vi "wait_with_status.vi"(4 "stat ref":refnum<vi>, 6 "stop ref":refnum<vi>, 7 "second stop ref":refnum<vi>, 8 "error in":errorcluster, 9 "comment":string, 10 "ignore error (False)":bool, 11 "ms to wait":i32) -> (0 "error out":errorcluster, 2 "Aborted?":bool)   [LabVIEW 2020, in "varilib.lvlib"]
doc: "Interruptable delay timer. It waits for given amount of milliseconds. When 'stop ref' is assigned with reference to boolean button it will terminate the delay when logical state of the boolean is True. If 'stat ref' is assigned with reference to string indicator and delay is over 1 second it will periodically write status string in following format:'Waiting 3 of 10 seconds%s' where %s is content of 'comment' input. When the wait loop is done the original content of 'stat ref' will be restored.\nThe second reference control is used to interrupt delay, however control is fully controlled by this VI: showing, reading and setting state, hiding."
uses:
  varilib.lvlib
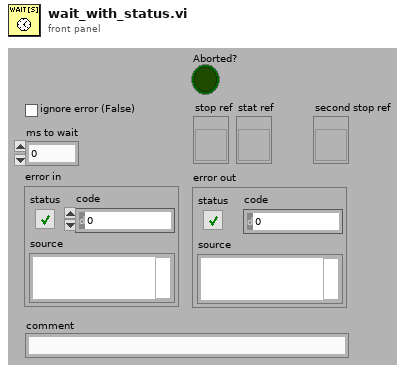
[diagram p1: front panel]
types:
  T1 = enum8{"Enabled", "Disabled", "Disabled and Grayed Out"}
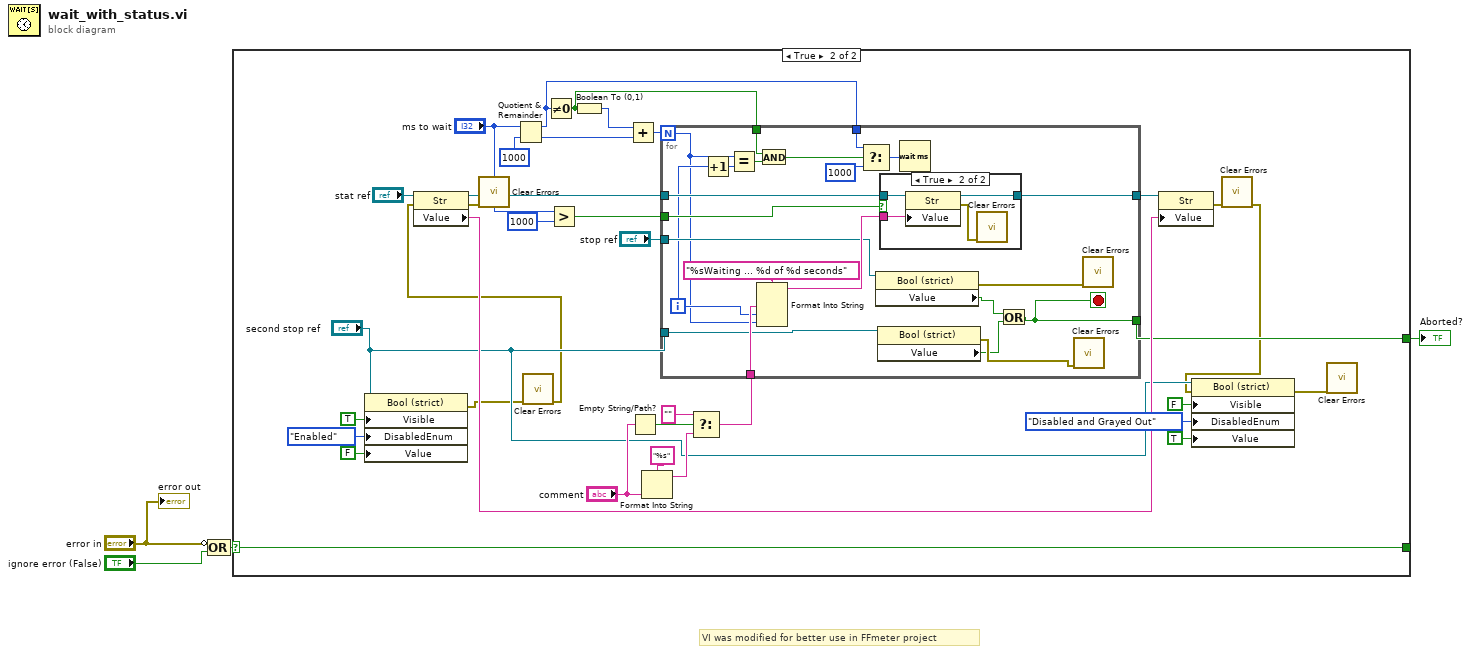
[diagram p0: block diagram]
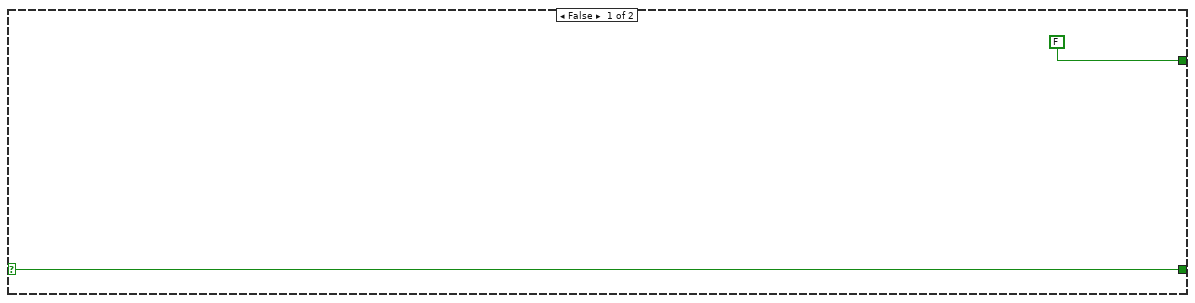
[diagram p2: hidden frame]
diagram:
  # "VI was modified for better use in FFmeter project"
  n1 = Compound Arithmetic op=OR(invert "error in", "ignore error (False)") -> (w2:bool)
  n2 = case shown="True" w2 {
    selector: w2 -> [w6 w25]
    tunnel: [w6 w25] -> _
    tunnel: [FALSE ("Value") w18] -> w1
    frame False {
    }
    frame True {
      n3 = property class="Bool (strict)"(reference="second stop ref", "Visible"=TRUE, "DisabledEnum"=T1."Enabled" ("Disabled"), "Value"=FALSE) -> (error out=w11:errorcluster)  [unwired: 1 in, 1 out]
      n4 = Quotient & Remainder(x="ms to wait", y=1000) -> (x-y*floor(x/y)=w31:i32, floor(x/y)=w32:i32)
      n5 = call <vilib>:"Clear Errors.vi"("error in (no error)"=w11) -> ("error out"=w10:errorcluster)  [unwired: 5 in, 1 out]
      n6 = property class="Str"(reference="stat ref", error in=w10) -> (reference out=w23:refnum<vi>, error out=w22:errorcluster, "Value"=w19:string)
      n7 = call <vilib>:"Clear Errors.vi"("error in (no error)"=w22) -> ()  [unwired: 5 in, 2 out]
      n8 = Not Equal To 0?(x=w31) -> (x != 0?=w30:bool)
      n9 = Greater?(x="ms to wait", y=1000) -> (0:w26:bool)
      n10 = Boolean To (0,1)(Boolean=w30) -> (0, 1=w29:i16)
      n11 = Add(x=w29, y=w32) -> (x+y=w33:i32)
      n12 = Empty String/Path?(string/path="comment") -> (empty?=w39:bool)
      n13 = Format Into String(format string="%s", "comment") -> (resulting string=w36:string)  [unwired: 2 in, 1 out]
      n14 = Select(t="", s=w39, f=w36) -> (s? t:f=w38:string)
      n15 = for {
        N: w33 -> [w47]
        tunnel: w23 -> [w63]
        tunnel: "stop ref" -> [w60]
        tunnel: w38 -> [w49]
        tunnel: w31 -> [w57]
        tunnel: w30 -> [w54]
        tunnel: w26 -> [w52]
        tunnel: [w50] -> w21
        tunnel: [w42] -> w18
        tunnel: "second stop ref" -> [w46]
        i -> [w48]
        stop <- w42 stop-if-true
        n16 = Increment(x=w48) -> (x+1=w56:i32)
        n17 = Equal?(x=w47, y=w56) -> (x = y?=w55:bool)
        n18 = Format Into String(format string="%sWaiting ... %d of %d seconds", w49, w48, w47) -> (resulting string=w62:string)  [unwired: 2 in, 1 out]
        n19 = And(x=w54, y=w55) -> (x .and. y?=w53:bool)
        n20 = Select(t=w57, s=w53, f=u32 1000 ("milliseconds to wait")) -> (s? t:f=w59:u32)
        n21 = property class="Bool (strict)"(reference=w60) -> (error out=w51:errorcluster, "Value"=w44:bool)  [unwired: 1 in, 1 out]
        n22 = property class="Bool (strict)"(reference=w46) -> (error out=w45:errorcluster, "Value"=w43:bool)  [unwired: 1 in, 1 out]
        n23 = case shown="True" w52 {
          tunnel: w63 -> [w64 w68]
          tunnel: w62 -> [_ w67]
          tunnel: [w64 w65] -> w50
          frame False {
          }
          frame True {
            n24 = property class="Str"(reference=w68, "Value"=w67) -> (reference out=w65:refnum<vi>, error out=w66:errorcluster)  [unwired: 1 in]
            n25 = call <vilib>:"Clear Errors.vi"("error in (no error)"=w66) -> ()  [unwired: 5 in, 2 out]
          }
        }
        n26 = Wait (ms)(milliseconds to wait=w59) -> ()  [unwired: 1 out]
        n27 = Or(x=w44, y=w43) -> (x .or. y?=w42:bool)
        n28 = call <vilib>:"Clear Errors.vi"("error in (no error)"=w45) -> ()  [unwired: 5 in, 2 out]
        n29 = call <vilib>:"Clear Errors.vi"("error in (no error)"=w51) -> ()  [unwired: 5 in, 2 out]
      }
      n30 = property class="Str"(reference=w21, "Value"=w19) -> (error out=w20:errorcluster)  [unwired: 1 in, 1 out]
      n31 = call <vilib>:"Clear Errors.vi"("error in (no error)"=w20) -> ("error out"=w14:errorcluster)  [unwired: 5 in, 1 out]
      n32 = property class="Bool (strict)"(reference="second stop ref", error in=w14, "Visible"=FALSE, "DisabledEnum"=T1."Disabled and Grayed Out" ("Disabled"), "Value"=TRUE) -> (error out=w13:errorcluster)  [unwired: 1 out]
      n33 = call <vilib>:"Clear Errors.vi"("error in (no error)"=w13) -> ()  [unwired: 5 in, 2 out]
    }
  }
  "Aborted?" <- w1
  "error out" <- "error in"
